vi "rszvl_core_global.vi"() -> ()   [LabVIEW 2014] (continued)
"Data Type"=4, "Access"=1, "Identifier"="RSZVL_ATTR_MARKER_SEARCH_PEAK", "Range Table"="", "Command"="CALC:MARK{Marker}:MAX", "Read Callback"="", "Write Callback"="", "Range Callback"="", "Check Callback"="", "Rngtable Callback"="", "Coerce Callback"="", "User Callback"="", "Supported Models"="", "Instrument Options"="", "Repeated Capabilities"="", "Restricted Repeated Capabilities"="", "Help"="This attribute positions the marker to the current maximum value of the corresponding trace. The corresponding marker is activated first or switched to the marker mode.\nNote: If no maximum value is found on the trace (level spacing to adjacent values < peak excursion), an execution error (error eode: -200) is produced.\n\nAvailable Repeated Capabilities:\nMarker: M1,M2,M3,M4\r\n\nRemote-control command(s):\nCALCulate<1|2>:MARKer<1 to 4>:MAXimum[:PEAK]", "Flags"={"OPC Wait"=FALSE, "Dont check status"=FALSE, "*WAI"=FALSE}, "Check Status Callback"=""}, {"Level"=3, "Descriptive Name"="Marker Search Peak Next Maximum", "Class Only"=FALSE, "Data Type"=4, "Access"=1, "Identifier"="RSZVL_ATTR_MARKER_SEARCH_PEAK_NEXT", "Range Table"="", "Command"="CALC:MARK{Marker}:MAX:NEXT", "Read Callback"="", "Write Callback"="", "Range Callback"="", "Check Callback"="", "Rngtable Callback"="", "Coerce Callback"="", "User Callback"="", "Supported Models"="", "Instrument Options"="", "Repeated Capabilities"="", "Restricted Repeated Capabilities"="", "Help"="This attribute positions the marker to the next smaller maximum value of the corresponding trace.\n\nNote: If no next smaller maximum value is found on the trace (level spacing to adjacent values < peak excursion), an execution error (error code: -200) is produced.\n\nAvailable Repeated Capabilities:\nMarker: M1,M2,M3,M4\r\n\nRemote-control command(s):\nCALCulate<1|2>:MARKer<1 to 4>:MAXimum:NEXT", "Flags"={"OPC Wait"=FALSE, "Dont check status"=FALSE, "*WAI"=FALSE}, "Check Status Callback"=""}, {"Level"=3, "Descriptive Name"="Marker Search Peak Right Maximum", "Class Only"=FALSE, "Data Type"=4, "Access"=1, "Identifier"="RSZVL_ATTR_MARKER_SEARCH_PEAK_RIGHT", "Range Table"="", "Command"="CALC:MARK{Marker}:MAX:RIGH", "Read Callback"="", "Write Callback"="", "Range Callback"="", "Check Callback"="", "Rngtable Callback"="", "Coerce Callback"="", "User Callback"="", "Supported Models"="", "Instrument Options"="", "Repeated Capabilities"="", "Restricted Repeated Capabilities"="", "Help"="This attribute positions the marker to the next smaller maximum value to the right of the current value (i.e. in ascending X values) on the corresponding trace.\n\nNote: If no next smaller maximum value is found on the trace (level spacing to adjacent values < peak excursion), an execution error (error code: -200) is produced.\n\nAvailable Repeated Capabilities:\nMarker: M1,M2,M3,M4\r\n\nRemote-control command(s):\nCALCulate<1|2>:MARKer<1 to 4>:MAXimum:RIGHt", "Flags"={"OPC Wait"=FALSE, "Dont check status"=FALSE, "*WAI"=FALSE}, "Check Status Callback"=""}, {"Level"=3, "Descriptive Name"="Marker Search Peak Left Maximum", "Class Only"=FALSE, "Data Type"=4, "Access"=1, "Identifier"="RSZVL_ATTR_MARKER_SEARCH_PEAK_LEFT", "Range Table"="", "Command"="CALC:MARK{Marker}:MAX:LEFT", "Read Callback"="", "Write Callback"="", "Range Callback"="", "Check Callback"="", "Rngtable Callback"="", "Coerce Callback"="", "User Callback"="", "Supported Models"="", "Instrument Options"="", "Repeated Capabilities"="", "Restricted Repeated Capabilities"="", "Help"="This attribute positions the marker to the next smaller maximum value to the left of the current value (i.e. in descending X values) on the trace.\n\nNote: If no next smaller maximum value is found on the trace (level spacing to adjacent values < peak excursion), an execution error (error code: -200) is produced.\n\nAvailable Repeated Capabilities:\nMarker: M1,M2,M3,M4\r\n\nRemote-control command(s):\nCALCulate<1|2>:MARKer<1 to 4>:MAXimum:LEFT", "Flags"={"OPC Wait"=FALSE, "Dont check status"=FALSE, "*WAI"=FALSE}, "Check Status Callback"=""}, {"Level"=3, "Descriptive Name"="Marker Search Peak Minimum", "Class Only"=FALSE, "Data Type"=4, "Access"=1, "Identifier"="RSZVL_ATTR_MARKER_SEARCH_MIN", "Range Table"="", "Command"="CALC:MARK{Marker}:MIN", "Read Callback"="", "Write Callback"="", "Range Callback"="", "Check Callback"="", "Rngtable Callback"="", "Coerce Callback"="", "User Callback"="", "Supported Models"="", "Instrument Options"="", "Repeated Capabilities"="", "Restricted Repeated Capabilities"="", "Help"="This attribute positions the marker to the current minimum value of the corresponding trace. The corresponding marker is activated first or switched to marker mode, if necessary.\n\nNote: If no minimum value is found on the trace (level spacing to adjacent values < peak excursion), an execution error (error code: -200) is produced.\n\nAvailable Repeated Capabilities:\nMarker: M1,M2,M3,M4\r\n\nRemote-control command(s):\nCALCulate<1|2>:MARKer<1 to 4>:MINimum[:PEAK]", "Flags"={"OPC Wait"=FALSE, "Dont check status"=FALSE, "*WAI"=FALSE}, "Check Status Callback"=""}, {"Level"=3, "Descriptive Name"="Marker Search Next Minimum", "Class Only"=FALSE, "Data Type"=4, "Access"=1, "Identifier"="RSZVL_ATTR_MARKER_SEARCH_MIN_NEXT", "Range Table"="", "Command"="CALC:MARK{Marker}:MIN:NEXT", "Read Callback"="", "Write Callback"="", "Range Callback"="", "Check Callback"="", "Rngtable Callback"="", "Coerce Callback"="", "User Callback"="", "Supported Models"="", "Instrument Options"="", "Repeated Capabilities"="", "Restricted Repeated Capabilities"="", "Help"="This attribute positions the marker to the next higher minimum value of the corresponding trace.\n\nNote: If no next higher minimum value is found on the trace (level spacing to adjacent values < peak excursion), an execution error (error code: -200) is produced.\n\nAvailable Repeated Capabilities:\nMarker: M1,M2,M3,M4\r\n\nRemote-control command(s):\nCALCulate<1|2>:MARKer<1 to 4>:MINimum:NEXT", "Flags"={"OPC Wait"=FALSE, "Dont check status"=FALSE, "*WAI"=FALSE}, "Check Status Callback"=""}, {"Level"=3, "Descriptive Name"="Marker Search Peak Maximum Auto", "Class Only"=FALSE, "Data Type"=3, "Access"=2, "Identifier"="RSZVL_ATTR_MARKER_SEARCH_PEAK_AUTO", "Range Table"="", "Command"="CALC:MARK:MAX:AUTO", "Read Callback"="", "Write Callback"="", "Range Callback"="", "Check Callback"="", "Rngtable Callback"="", "Coerce Callback"="", "User Callback"="", "Supported Models"="", "Instrument Options"="", "Repeated Capabilities"="", "Restricted Repeated Capabilities"="", "Help"="This attribute switches an automatic maximum peak search for marker 1 at the end of each particular sweep on and off. The actual marker search limit settings (LEFT LIMIT, RIGHT LIMIT, THRESHOLD, EXCLUDE LO) are taken into account.\n\nAvailable Repeated Capabilities:\nNone\n\nRemote-control command(s):\nCALCulate<1|2>:MARKer<1...4>:MAXimum:AUTO", "Flags"={"OPC Wait"=FALSE, "Dont check status"=FALSE, "*WAI"=FALSE}, "Check Status Callback"=""}, {"Level"=3, "Descriptive Name"="Marker Search Minimum Auto", "Class Only"=FALSE, "Data Type"=3, "Access"=2, "Identifier"="RSZVL_ATTR_MARKER_SEARCH_MIN_AUTO", "Range Table"="", "Command"="CALC:MARK:MIN:AUTO", "Read Callback"="", "Write Callback"="", "Range Callback"="", "Check Callback"="", "Rngtable Callback"="", "Coerce Callback"="", "User Callback"="", "Supported Models"="", "Instrument Options"="", "Repeated Capabilities"="", "Restricted Repeated Capabilities"="", "Help"="This attribute switches an automatic minimum peak search for marker 1 at the end of each particular sweep on and off. The actual marker search limit settings (LEFT LIMIT, RIGHT LIMIT, THRESHOLD, EXCLUDE LO) are taken into account.\n\nAvailable Repeated Capabilities:\nNone\n\nRemote-control command(s):\nCALCulate<1|2>:MARKer<1...4>:MINimum:AUTO", "Flags"={"OPC Wait"=FALSE, "Dont check status"=FALSE, "*WAI"=FALSE}, "Check Status Callback"=""}, {"Level"=2, "Descriptive Name"="Marker Search Configuration", "Class Only"=TRUE, "Data Type"=0, "Access"=0, "Identifier"="", "Range Table"="", "Command"="", "Read Callback"="", "Write Callback"="", "Range Callback"="", "Check Callback"="", "Rngtable Callback"="", "Coerce Callback"="", "User Callback"="", "Supported Models"="", "Instrument Options"="", "Repeated Capabilities"="", "Restricted Repeated Capabilities"="", "Help"="Configures marker search parameters.\n\n(1) Marker Threshold State:\nThis attribute switches on or off the threshold line. The unit depends on the setting performed with CALC:UNIT.\n\n(2) Marker Threshold:\nThis attribute defines the threshold value for the maximum/minimum search of markers with marker search functions MAX PEAK, NEXT PEAK, etc. The associated display line is automatically switched on.\n\n(3) Marker Peak Excursion:\nThis attribute defines the peak excursion., i.e. the spacing below a trace maximum which must be attained before a new maximum is recognized, or the spacing above a trace minimum which must be attained before a new minimum is recognized. The set value is valid for all markers and delta markers. The unit depends on the selected operating mode.\n\n(4) Marker Search Limits State:\nThis attribute switches between a limited (ON) and unlimited (OFF) search range. The function is independent of the selection of a marker.\n\n(5) Marker Search Limits Left:\nThis attribute sets the left limit of the search range for markers and delta markers. Depending on the x axis domain the indicated value defines a frequency (span > 0) or time (span = 0). The function is independent of the selection of a marker.\n\n(6) Marker Search Limits Right:\nThis attribute sets the right limit of the search range for markers and delta markers. Depending on the x axis domain the indicated value defines a frequency (span > 0) or time (span = 0). The function is independent of the selection of a marker.", "Flags"={"OPC Wait"=FALSE, "Dont check status"=FALSE, "*WAI"=FALSE}, "Check Status Callback"=""}, {"Level"=3, "Descriptive Name"="Marker Threshold State", "Class Only"=FALSE, "Data Type"=3, "Access"=2, "Identifier"="RSZVL_ATTR_MARKER_THRESHOLD_STATE", "Range Table"="", "Command"="CALC:THR:STAT", "Read Callback"="", "Write Callback"="", "Range Callback"="", "Check Callback"="", "Rngtable Callback"="", "Coerce Callback"="", "User Callback"="", "Supported Models"="", "Instrument Options"="", "Repeated Capabilities"="", "Restricted Repeated Capabilities"="", "Help"="This attribute switches on or off the threshold line. The unit depends on the setting performed with CALC:UNIT.\n\nAvailable Repeated Capabilities:\nNone\n\nRemote-control command(s):\nCALCulate<1|2>:THReshold:STATe ON | OFF", "Flags"={"OPC Wait"=FALSE, "Dont check status"=FALSE, "*WAI"=FALSE}, "Check Status Callback"=""}, {"Level"=3, "Descriptive Name"="Marker Threshold", "Class Only"=FALSE, "Data Type"=1, "Access"=2, "Identifier"="RSZVL_ATTR_MARKER_THRESHOLD", "Range Table"="", "Command"="CALC:THR", "Read Callback"="", "Write Callback"="", "Range Callback"="", "Check Callback"="", "Rngtable Callback"="", "Coerce Callback"="", "User Callback"="", "Supported Models"="", "Instrument Options"="", "Repeated Capabilities"="", "Restricted Repeated Capabilities"="", "Help"="This attribute defines the threshold value for the maximum/minimum search of markers with marker search functions MAX PEAK, NEXT PEAK, etc. The associated display line is automatically switched on.\n\nAvailable Repeated Capabilities:\nNone\n\nRemote-control command(s):\nCALCulate<1|2>:THReshold", "Flags"={"OPC Wait"=FALSE, "Dont check status"=FALSE, "*WAI"=FALSE}, "Check Status Callback"=""}, {"Level"=3, "Descriptive Name"="Marker Peak Excursion", "Class Only"=FALSE, "Data Type"=1, "Access"=2, "Identifier"="RSZVL_ATTR_PEAK_EXCURSION", "Range Table"="", "Command"="CALC:MARK:PEXC", "Read Callback"="", "Write Callback"="", "Range Callback"="", "Check Callback"="", "Rngtable Callback"="", "Coerce Callback"="", "User Callback"="", "Supported Models"="", "Instrument Options"="", "Repeated Capabilities"="", "Restricted Repeated Capabilities"="", "Help"="This attribute defines the peak excursion., i.e. the spacing below a trace maximum which must be attained before a new maximum is recognized, or the spacing above a trace minimum which must be attained before a new minimum is recognized. The set value is valid for all markers and delta markers. The unit depends on the selected operating mode.\n\nAvailable Repeated Capabilities:\nNone\n\nRemote-control command(s):\nCALCulate<1|2>:MARKer<1 to 4>:PEXCursion", "Flags"={"OPC Wait"=FALSE, "Dont check status"=FALSE, "*WAI"=FALSE}, "Check Status Callback"=""}, {"Level"=3, "Descriptive Name"="Marker Search Limits State", "Class Only"=FALSE, "Data Type"=3, "Access"=2, "Identifier"="RSZVL_ATTR_MARKER_SEARCH_LIMITS_STATE", "Range Table"="", "Command"="CALC:MARK:X:SLIM", "Read Callback"="", "Write Callback"="", "Range Callback"="", "Check Callback"="", "Rngtable Callback"="", "Coerce Callback"="", "User Callback"="", "Supported Models"="", "Instrument Options"="", "Repeated Capabilities"="", "Restricted Repeated Capabilities"="", "Help"="This attribute switches between a limited (ON) and unlimited (OFF) search range. The function is independent of the selection of a marker.\n\nAvailable Repeated Capabilities:\nNone\n\nRemote-control command(s):\nCALCulate<1|2>:MARKer<1 to 4>:X:SLIMits[:STATe] ON | OFF", "Flags"={"OPC Wait"=FALSE, "Dont check status"=FALSE, "*WAI"=FALSE}, "Check Status Callback"=""}, {"Level"=3, "Descriptive Name"="Marker Search Limits Left", "Class Only"=FALSE, "Data Type"=1, "Access"=2, "Identifier"="RSZVL_ATTR_MARKER_SEARCH_LIMITS_LEFT", "Range Table"="", "Command"="CALC:MARK:X:SLIM:LEFT", "Read Callback"="", "Write Callback"="", "Range Callback"="", "Check Callback"="", "Rngtable Callback"="", "Coerce Callback"="", "User Callback"="", "Supported Models"="", "Instrument Options"="", "Repeated Capabilities"="", "Restricted Repeated Capabilities"="", "Help"="This attribute sets the left limit of the search range for markers and delta markers. Depending on the x axis domain the indicated value defines a frequency (span > 0) or time (span = 0). The function is independent of the selection of a marker.\n\nAvailable Repeated Capabilities:\nNone\n\nRemote-control command(s):\nCALCulate<1|2>:MARKer<1 to 4>:X:SLIMits:LEFT", "Flags"={"OPC Wait"=FALSE, "Dont check status"=FALSE, "*WAI"=FALSE}, "Check Status Callback"=""}, {"Level"=3, "Descriptive Name"="Marker Search Limits Right", "Class Only"=FALSE, "Data Type"=1, "Access"=2, "Identifier"="RSZVL_ATTR_MARKER_SEARCH_LIMITS_RIGHT", "Range Table"="", "Command"="CALC:MARK:X:SLIM:RIGHT", "Read Callback"="", "Write Callback"="", "Range Callback"="", "Check Callback"="", "Rngtable Callback"="", "Coerce Callback"="", "User Callback"="", "Supported Models"="", "Instrument Options"="", "Repeated Capabilities"="", "Restricted Repeated Capabilities"="", "Help"="This attribute sets the right limit of the search range for markers and delta markers. Depending on the x axis domain the indicated value defines a frequency (span > 0) or time (span = 0). The function is independent of the selection of a marker.\n\nAvailable Repeated Capabilities:\nNone\n\nRemote-control command(s):\nCALCulate<1|2>:MARKer<1 to 4>:X:SLIMits:RIGHT", "Flags"={"OPC Wait"=FALSE, "Dont check status"=FALSE, "*WAI"=FALSE}, "Check Status Callback"=""}, {"Level"=2, "Descriptive Name"="Marker Functions", "Class Only"=TRUE, "Data Type"=0, "Access"=0, "Identifier"="", "Range Table"="", "Command"="", "Read Callback"="", "Write Callback"="", "Range Callback"="", "Check Callback"="", "Rngtable Callback"="", "Coerce Callback"="", "User Callback"="", "Supported Models"="", "Instrument Options"="", "Repeated Capabilities"="", "Restricted Repeated Capabilities"="", "Help"="Marker Functions.\n\n(1) Marker Peak List Count:\nThis attribute searches the selected trace for the indicated number of maxima. The number of maxima found depends on the waveform and value set for the Peak Excursion parameter, however, a maximum number of 50 maxima are determined. Only the signals which exceed their surrounding values at least by the value indicated by the peak excursion parameter will be recognized as maxima. Therefore, the number of maxima found is not automatically the same as the number of maxima desired.\n\n(2) Marker Peak List Found:\nThis attribute reads out the number of maxima found during the search. If no search for maxima has been performed, 0 is returned.\n\n(3) Marker Peak List Sort:\nThis attribute sets the sort mode for the search for maxima.\n\n(4) Marker Zoom:\nThis attribute defines the range to be zoomed around marker 1. Marker 1 is activated first, if necessary.\nThe subsequent frequency sweep is stopped at the marker position and the frequency of the signal is counted. This frequency becomes the new center frequency, and the zoomed span is set. In order to recognize the end of the operation the synchronization to the sweep end should be activated. This is only possible in single sweep mode.\n\n(5) Marker Demodulation State:\nThis attribute switches on or off the audio demodulator when the indicated marker is reached. In the frequency domain (span > 0) the hold time can be defined at the corresponding marker position with RSZVL_ATTR_MARKER_DEMOD_HOLDOFF.\nIn the time domain (span = 0) the demodulation is permanently active.\n\n(6) Marker Demodulation Type:\nThis attribute selects the demodulation type for the audio demodulator.\n\n(7) Marker Demodulation Holdoff:\nThis attribute defines the hold time at the marker position for the demodulation in the frequency domain (span > 0).\n\n(8) Marker Demodulation Continuous:\nThis attribute switches on or off the continuous demodulation in the frequency domain (span >0). Thus acoustic monitoring of the signals can be performed in the frequency domain. The function does not depend on the selected marker.\n\n(9) Marker To Center:\nThis attribute sets the center frequency equal to the frequency of the indicated marker.\nIf marker 2, 3 or 4 is selected and used as delta marker, it is switched to the marker mode.\n\n(10) Marker To Step Width:\nThis attribute sets the step width of the center frequency to the X value of the current marker. If marker 2, 3 or 4 is selected and used as delta marker, it is switched to the marker mode.\n\n(11) Marker To Reference:\nThis attribute sets the reference level to the power measured by the indicated marker. If marker 2, 3 or 4 is selected and used as delta marker, it is switched to marker mode.\n\n(12) Marker Fixed Reference State:\nThis attribute switches the relative measurement to a fixed reference value on or off. Marker 1 will be activated previously and a peak search will be performed, if necessary. If marker 1 is activated, its position becomes the reference point for the measurement. The reference point can then be modified with commands CALCulate:DELTamarker:FUNCtion:FIXed:RPOint:X and to :RPOint:Y independently of the position of marker 1 and of a trace. It is valid for all delta markers as long as the function is active.\n\n(13) Marker Fixed Ref Point Level:\nThis attribute defines a new reference point level for all delta markers for a measurement with fixed reference point.\n(CALCulate:DELTamarker:FUNCtion:FIXed:STATe ON).\nFor phase-noise measurements (CALCulate:DELTamarker:FUNCtion:PNOise:STATe ON), the command defines a new reference point level for delta marker 2.\n\n(14) Marker Fixed Ref Point Level Offset:\nThis attribute defines an additional level offset for the measurement with fixed reference value (CALCulate:DELTamarker:FUNCtion:FIXed:STATe ON). For this measurement, the offset is included in the display of all delta markers.\nFor phase-noise measurements (CALCulate:DELTamarker:FUNCtion:PNOise:STATe ON), the command defines an additional level offset which is included in the display of delta marker 2.\n\n(15) Marker Fixed Ref Point Frequency:\nThis attribute defines a new reference frequency (span > 0) or time (span = 0) for all delta markers for a measurement with fixed reference value (CALCulate:DELTamarker:FUNCtion:FIXed:STATe ON).\nFor phase-noise measurements (CALCulate:DELTamarker:FUNCtion:PNOise:STATe ON), the command defines a new reference frequency or time for delta marker 2.\n\n(16) Marker Fixed Ref Point Peak Search:\nThis attribute sets the reference point level for all delta markers for a measurement with fixed reference point (CALC:DELT:FUNC:FIX:STAT ON) to the peak of the selected trace.", "Flags"={"OPC Wait"=FALSE, "Dont check status"=FALSE, "*WAI"=FALSE}, "Check Status Callback"=""}, {"Level"=3, "Descriptive Name"="Marker Peak List Count", "Class Only"=FALSE, "Data Type"=0, "Access"=2, "Identifier"="RSZVL_ATTR_MARKER_PEAK_LIST_COUNT", "Range Table"="rszvl_rngMarkerPeakListCount", "Command"="CALC:MARK{Marker}:FUNC:FPE", "Read Callback"="", "Write Callback"="", "Range Callback"="", "Check Callback"="", "Rngtable Callback"="", "Coerce Callback"="", "User Callback"="", "Supported Models"="", "Instrument Options"="", "Repeated Capabilities"="", "Restricted Repeated Capabilities"="", "Help"="This attribute searches the selected trace for the indicated number of maxima. The number of maxima found depends on the waveform and value set for the Peak Excursion parameter, however, a maximum number of 50 maxima are determined. Only the signals which exceed their surrounding values at least by the value indicated by the peak excursion parameter will be recognized as maxima. Therefore, the number of maxima found is not automatically the same as the number of maxima desired.\n\nAvailable Repeated Capabilities:\nMarker: M1,M2,M3,M4\r\n\nRemote-control command(s):\nCALCulate<1|2>:MARKer<1 to 4>:FUNCtion:FPEaks[:IMMediate]", "Flags"={"OPC Wait"=FALSE, "Dont check status"=FALSE, "*WAI"=FALSE}, "Check Status Callback"=""}, {"Level"=3, "Descriptive Name"="Marker Peak List Found", "Class Only"=FALSE, "Data Type"=0, "Access"=0, "Identifier"="RSZVL_ATTR_MARKER_PEAK_LIST_FOUND", "Range Table"="", "Command"="CALC:MARK{Marker}:FUNC:FPE:COUN?", "Read Callback"="", "Write Callback"="", "Range Callback"="", "Check Callback"="", "Rngtable Callback"="", "Coerce Callback"="", "User Callback"="", "Supported Models"="", "Instrument Options"="", "Repeated Capabilities"="", "Restricted Repeated Capabilities"="", "Help"="This attribute reads out the number of maxima found during the search. If no search for maxima has been performed, 0 is returned.\n\nAvailable Repeated Capabilities:\nMarker: M1,M2,M3,M4\r\n\nRemote-control command(s):\nCALCulate<1|2>:MARKer<1 to 4>:FUNCtion:FPEaks:COUNt?", "Flags"={"OPC Wait"=FALSE, "Dont check status"=FALSE, "*WAI"=FALSE}, "Check Status Callback"=""}, {"Level"=3, "Descriptive Name"="Marker Peak List Sort", "Class Only"=FALSE, "Data Type"=0, "Access"=2, "Identifier"="RSZVL_ATTR_MARKER_PEAK_LIST_SORT", "Range Table"="rszvl_rngMarkerPeakListSort", "Command"="CALC:MARK{Marker}:FUNC:FPE:SORT", "Read Callback"="", "Write Callback"="", "Range Callback"="", "Check Callback"="", "Rngtable Callback"="", "Coerce Callback"="", "User Callback"="", "Supported Models"="", "Instrument Options"="", "Repeated Capabilities"="", "Restricted Repeated Capabilities"="", "Help"="This attribute sets the sort mode for the search for maxima.\n\nAvailable Repeated Capabilities:\nMarker: M1,M2,M3,M4\r\n\nRemote-control command(s):\nCALCulate<1|2>:MARKer<1 to 4>:FUNCtion:FPEaks:SORT X | Y", "Flags"={"OPC Wait"=FALSE, "Dont check status"=FALSE, "*WAI"=FALSE}, "Check Status Callback"=""}, {"Level"=3, "Descriptive Name"="Marker Zoom", "Class Only"=FALSE, "Data Type"=1, "Access"=2, "Identifier"="RSZVL_ATTR_MARKER_ZOOM", "Range Table"="", "Command"="CALC:MARK:FUNC:ZOOM", "Read Callback"="", "Write Callback"="", "Range Callback"="", "Check Callback"="", "Rngtable Callback"="", "Coerce Callback"="", "User Callback"="", "Supported Models"="", "Instrument Options"="", "Repeated Capabilities"="", "Restricted Repeated Capabilities"="", "Help"="This attribute defines the range to be zoomed around marker 1. Marker 1 is activated first, if necessary.\nThe subsequent frequency sweep is stopped at the marker position and the frequency of the signal is counted. This frequency becomes the new center frequency, and the zoomed span is set. In order to recognize the end of the operation the synchronization to the sweep end should be activated. This is only possible in single sweep mode.\n\nAvailable Repeated Capabilities:\nNone\n\nRemote-control command(s):\nCALCulate<1|2>:MARKer<1 to 4>:FUNCtion:ZOOM", "Flags"={"OPC Wait"=TRUE, "Dont check status"=FALSE, "*WAI"=FALSE}, "Check Status Callback"=""}, {"Level"=3, "Descriptive Name"="Marker Demodulation State", "Class Only"=FALSE, "Data Type"=3, "Access"=2, "Identifier"="RSZVL_ATTR_MARKER_DEMOD_STATE", "Range Table"="", "Command"="CALC:MARK{Marker}:FUNC:DEM", "Read Callback"="", "Write Callback"="", "Range Callback"="", "Check Callback"="", "Rngtable Callback"="", "Coerce Callback"="", "User Callback"="", "Supported Models"="", "Instrument Options"="", "Repeated Capabilities"="", "Restricted Repeated Capabilities"="", "Help"="This attribute switches on or off the audio demodulator when the indicated marker is reached. In the frequency domain (span > 0) the hold time can be defined at the corresponding marker position with RSZVL_ATTR_MARKER_DEMOD_HOLDOFF.\nIn the time domain (span = 0) the demodulation is permanently active.\n\nAvailable Repeated Capabilities:\nMarker: M1,M2,M3,M4\r\n\nRemote-control command(s):\nCALCulate<1|2>:MARKer<1 to 4>:FUNCtion:DEModulation[:STATe] ON | OFF", "Flags"={"OPC Wait"=FALSE, "Dont check status"=FALSE, "*WAI"=FALSE}, "Check Status Callback"=""}, {"Level"=3, "Descriptive Name"="Marker Demodulation Type", "Class Only"=FALSE, "Data Type"=0, "Access"=2, "Identifier"="RSZVL_ATTR_MARKER_DEMOD_TYPE", "Range Table"="rszvl_rngMarkerDemodType", "Command"="CALC:MARK:FUNC:DEM:SEL", "Read Callback"="", "Write Callback"="", "Range Callback"="", "Check Callback"="", "Rngtable Callback"="", "Coerce Callback"="", "User Callback"="", "Supported Models"="", "Instrument Options"="", "Repeated Capabilities"="", "Restricted Repeated Capabilities"="", "Help"="This attribute selects the demodulation type for the audio demodulator.\n\nAvailable Repeated Capabilities:\nNone\n\nRemote-control command(s):\nCALCulate<1|2>:MARKer<1 to 4>:FUNCtion:DEModulation:SELect AM | FM", "Flags"={"OPC Wait"=FALSE, "Dont check status"=FALSE, "*WAI"=FALSE}, "Check Status Callback"=""}, {"Level"=3, "Descriptive Name"="Marker Demodulation Holdoff", "Class Only"=FALSE, "Data Type"=1, "Access"=2, "Identifier"="RSZVL_ATTR_MARKER_DEMOD_HOLDOFF", "Range Table"="rszvl_rngMarkerDemodHoldoff", "Command"="CALC:MARK:FUNC:DEM:HOLD", "Read Callback"="", "Write Callback"="", "Range Callback"="", "Check Callback"="", "Rngtable Callback"="", "Coerce Callback"="", "User Callback"="", "Supported Models"="", "Instrument Options"="", "Repeated Capabilities"="", "Restricted Repeated Capabilities"="", "Help"="This attribute defines the hold time at the marker position for the demodulation in the frequency domain (span > 0).\n\nAvailable Repeated Capabilities:\nNone\n\nRemote-control command(s):\nCALCulate<1|2>:MARKer<1 to 4>:FUNCtion:DEModulation:HOLDoff", "Flags"={"OPC Wait"=FALSE, "Dont check status"=FALSE, "*WAI"=FALSE}, "Check Status Callback"=""}, {"Level"=3, "Descriptive Name"="Marker Demodulation Continuous", "Class Only"=FALSE, "Data Type"=3, "Access"=2, "Identifier"="RSZVL_ATTR_MARKER_DEMOD_CONT", "Range Table"="", "Command"="CALC:MARK:FUNC:DEM:CONT", "Read Callback"="", "Write Callback"="", "Range Callback"="", "Check Callback"="", "Rngtable Callback"="", "Coerce Callback"="", "User Callback"="", "Supported Models"="", "Instrument Options"="", "Repeated Capabilities"="", "Restricted Repeated Capabilities"="", "Help"="This attribute switches on or off the continuous demodulation in the frequency domain (span >0). Thus acoustic monitoring of the signals can be performed in the frequency domain. The function does not depend on the selected marker.\n\nAvailable Repeated Capabilities:\nNone\n\nRemote-control command(s):\nCALCulate<1|2>:MARKer<1 to 4>:FUNCtion:DEModulation:CONTinuous ON | OFF", "Flags"={"OPC Wait"=FALSE, "Dont check status"=FALSE, "*WAI"=FALSE}, "Check Status Callback"=""}, {"Level"=3, "Descriptive Name"="Marker To Center", "Class Only"=FALSE, "Data Type"=4, "Access"=1, "Identifier"="RSZVL_ATTR_MARKER_TO_CENTER", "Range Table"="", "Command"="CALC:MARK{Marker}:FUNC:CENT", "Read Callback"="", "Write Callback"="", "Range Callback"="", "Check Callback"="", "Rngtable Callback"="", "Coerce Callback"="", "User Callback"="", "Supported Models"="", "Instrument Options"="", "Repeated Capabilities"="", "Restricted Repeated Capabilities"="", "Help"="This attribute sets the center frequency equal to the frequency of the indicated marker.\nIf marker 2, 3 or 4 is selected and used as delta marker, it is switched to the marker mode.\n\nAvailable Repeated Capabilities:\nMarker: M1,M2,M3,M4\r\n\nRemote-control command(s):\nCALCulate<1|2>:MARKer<1 to 4>:FUNCtion:CENTer", "Flags"={"OPC Wait"=FALSE, "Dont check status"=FALSE, "*WAI"=FALSE}, "Check Status Callback"=""}, {"Level"=3, "Descriptive Name"="Marker To Step Width", "Class Only"=FALSE, "Data Type"=4, "Access"=1, "Identifier"="RSZVL_ATTR_MARKER_TO_STEP", "Range Table"="", "Command"="CALC:MARK{Marker}:FUNC:CST", "Read Callback"="", "Write Callback"="", "Range Callback"="", "Check Callback"="", "Rngtable Callback"="", "Coerce Callback"="", "User Callback"="", "Supported Models"="", "Instrument Options"="", "Repeated Capabilities"="", "Restricted Repeated Capabilities"="", "Help"="This attribute sets the step width of the center frequency to the X value of the current marker. If marker 2, 3 or 4 is selected and used as delta marker, it is switched to the marker mode.\n\nAvailable Repeated Capabilities:\nMarker: M1,M2,M3,M4\r\n\nRemote-control command(s):\nCALCulate<1|2>:MARKer<1 to 4>:FUNCtion:CSTep", "Flags"={"OPC Wait"=FALSE, "Dont check status"=FALSE, "*WAI"=FALSE}, "Check Status Callback"=""}, {"Level"=3, "Descriptive Name"="Marker To Reference", "Class Only"=FALSE, "Data Type"=4, "Access"=1, "Identifier"="RSZVL_ATTR_MARKER_TO_REFERENCE", "Range Table"="", "Command"="CALC:MARK{Marker}:FUNC:REF", "Read Callback"="", "Write Callback"="", "Range Callback"="", "Check Callback"="", "Rngtable Callback"="", "Coerce Callback"="", "User Callback"="", "Supported Models"="", "Instrument Options"="", "Repeated Capabilities"="", "Restricted Repeated Capabilities"="", "Help"="This attribute sets the reference level to the power measured by the indicated marker. If marker 2, 3 or 4 is selected and used as delta marker, it is switched to marker mode.\n\nAvailable Repeated Capabilities:\nMarker: M1,M2,M3,M4\r\n\nRemote-control command(s):\nCALCulate<1|2>:MARKer<1 to 4>:FUNCtion:REFerence", "Flags"={"OPC Wait"=FALSE, "Dont check status"=FALSE, "*WAI"=FALSE}, "Check Status Callback"=""}, {"Level"=3, "Descriptive Name"="Marker Fixed Reference State", "Class Only"=FALSE, "Data Type"=3, "Access"=2, "Identifier"="RSZVL_ATTR_MARKER_REF_STATE", "Range Table"="", "Command"="CALC:DELT:FUNC:FIX", "Read Callback"="", "Write Callback"="", "Range Callback"="", "Check Callback"="", "Rngtable Callback"="", "Coerce Callback"="", "User Callback"="", "Supported Models"="", "Instrument Options"="", "Repeated Capabilities"="", "Restricted Repeated Capabilities"="", "Help"="This attribute switches the relative measurement to a fixed reference value on or off. Marker 1 will be activated previously and a peak search will be performed, if necessary. If marker 1 is activated, its position becomes the reference point for the measurement. The reference point can then be modified with commands CALCulate:DELTamarker:FUNCtion:FIXed:RPOint:X and to :RPOint:Y independently of the position of marker 1 and of a trace. It is valid for all delta markers as long as the function is active.\n\nAvailable Repeated Capabilities:\nNone\n\nRemote-control command(s):\nCALCulate<1|2>:DELTamarker<1 to 4>:FUNCtion:FIXed[:STATe] ON | OFF", "Flags"={"OPC Wait"=FALSE, "Dont check status"=FALSE, "*WAI"=FALSE}, "Check Status Callback"=""}, {"Level"=3, "Descriptive Name"="Marker Fixed Ref Point Level", "Class Only"=FALSE, "Data Type"=1, "Access"=2, "Identifier"="RSZVL_ATTR_MARKER_REF_LEVEL", "Range Table"="rszvl_rngRefLevel", "Command"="CALC:DELT:FUNC:FIX:RPO:Y", "Read Callback"="", "Write Callback"="", "Range Callback"="", "Check Callback"="", "Rngtable Callback"="", "Coerce Callback"="", "User Callback"="", "Supported Models"="", "Instrument Options"="", "Repeated Capabilities"="", "Restricted Repeated Capabilities"="", "Help"="This attribute defines a new reference point level for all delta markers for a measurement with fixed reference point.\n(CALCulate:DELTamarker:FUNCtion:FIXed:STATe ON).\nFor phase-noise measurements (CALCulate:DELTamarker:FUNCtion:PNOise:STATe ON), the command defines a new reference point level for delta marker 2.\n\nAvailable Repeated Capabilities:\nNone\n\nRemote-control command(s):\nCALCulate<1|2>:DELTamarker<1 to 4>:FUNCtion:FIXed:RPOint:Y", "Flags"={"OPC Wait"=FALSE, "Dont check status"=FALSE, "*WAI"=FALSE}, "Check Status Callback"=""}, {"Level"=3, "Descriptive Name"="Marker Fixed Ref Point Level Offset", "Class Only"=FALSE, "Data Type"=1, "Access"=2, "Identifier"="RSZVL_ATTR_MARKER_REF_LEVEL_OFFSET", "Range Table"="rszvl_rngRefLevelOffset", "Command"="CALC:DELT:FUNC:FIX:RPO:Y:OFFS", "Read Callback"="", "Write Callback"="", "Range Callback"="", "Check Callback"="", "Rngtable Callback"="", "Coerce Callback"="", "User Callback"="", "Supported Models"="", "Instrument Options"="", "Repeated Capabilities"="", "Restricted Repeated Capabilities"="", "Help"="This attribute defines an additional level offset for the measurement with fixed reference value (CALCulate:DELTamarker:FUNCtion:FIXed:STATe ON). For this measurement, the offset is included in the display of all delta markers.\nFor phase-noise measurements (CALCulate:DELTamarker:FUNCtion:PNOise:STATe ON), the command defines an additional level offset which is included in the display of delta marker 2.\n\nAvailable Repeated Capabilities:\nNone\n\nRemote-control command(s):\nCALCulate<1|2>:DELTamarker<1 to 4>:FUNCtion:FIXed:RPOint:Y:OFFSet", "Flags"={"OPC Wait"=FALSE, "Dont check status"=FALSE, "*WAI"=FALSE}, "Check Status Callback"=""}, {"Level"=3, "Descriptive Name"="Marker Fixed Ref Point Frequency", "Class Only"=FALSE, "Data Type"=1, "Access"=2, "Identifier"="RSZVL_ATTR_MARKER_REF_FREQ", "Range Table"="", "Command"="CALC:DELT:FUNC:FIX:RPO:X", "Read Callback"="", "Write Callback"="", "Range Callback"="", "Check Callback"="", "Rngtable Callback"="", "Coerce Callback"="", "User Callback"="", "Supported Models"="", "Instrument Options"="", "Repeated Capabilities"="", "Restricted Repeated Capabilities"="", "Help"="This attribute defines a new reference frequency (span > 0) or time (span = 0) for all delta markers for a measurement with fixed reference value (CALCulate:DELTamarker:FUNCtion:FIXed:STATe ON).\nFor phase-noise measurements (CALCulate:DELTamarker:FUNCtion:PNOise:STATe ON), the command defines a new reference frequency or time for delta marker 2.\n\nAvailable Repeated Capabilities:\nNone\n\nRemote-control command(s):\nCALCulate<1|2>:DELTamarker<1 to 4>:FUNCtion:FIXed:RPOint:X", "Flags"={"OPC Wait"=FALSE, "Dont check status"=FALSE, "*WAI"=FALSE}, "Check Status Callback"=""}, {"Level"=3, "Descriptive Name"="Marker Fixed Ref Point Peak Search", "Class Only"=FALSE, "Data Type"=4, "Access"=1, "Identifier"="RSZVL_ATTR_MARKER_REF_PEAK", "Range Table"="", "Command"="CALC:DELT:FUNC:FIX:RPO:MAX", "Read Callback"="", "Write Callback"="", "Range Callback"="", "Check Callback"="", "Rngtable Callback"="", "Coerce Callback"="", "User Callback"="", "Supported Models"="", "Instrument Options"="", "Repeated Capabilities"="", "Restricted Repeated Capabilities"="", "Help"="This attribute sets the reference point level for all delta markers for a measurement with fixed reference point (CALC:DELT:FUNC:FIX:STAT ON) to the peak of the selected trace.\n\nAvailable Repeated Capabilities:\nNone\n\nRemote-control command(s):\nCALCulate<1|2>:DELTamarker<1 to 4>:FUNCtion:FIXed:RPOint:MAXimum[:PEAK]", "Flags"={"OPC Wait"=FALSE, "Dont check status"=FALSE, "*WAI"=FALSE}, "Check Status Callback"=""}, {"Level"=2, "Descriptive Name"="Delta Marker", "Class Only"=TRUE, "Data Type"=0, "Access"=0, "Identifier"="", "Range Table"="", "Command"="", "Read Callback"="", "Write Callback"="", "Range Callback"="", "Check Callback"="", "Rngtable Callback"="", "Coerce Callback"="", "User Callback"="", "Supported Models"="", "Instrument Options"="", "Repeated Capabilities"="", "Restricted Repeated Capabilities"="", "Help"="Delta Marker attributes configuration.\n\n(1) Delta Marker State:\nThis attribute switches on and off the delta marker when delta marker 1 is selected. The corresponding marker becomes the delta marker when delta marker 2 to 4 is selected. If the corresponding marker is not activated, it will be activated and positioned on  the maximum of the measurement curve.\n\n(2) Delta Marker Mode:\nThis attribute switches between relative and absolute frequency input of the delta marker (or time with span = 0). It affects all delta markers.\nRepeated capabilitiy Delta Marker are used to prevent switching On Delta Marker 1, if the user uses Delta Marker 2.\n\n(3) Delta Marker Position:\nThis attribute positions the selected delta marker to the indicated frequency (span > 0), time (span = 0) or level (APD measurement = ON or CCDFmeasurement = ON). The input is in absolute values or relative to marker 1 depending on the attribute RSZVL_ATTR_REFERENCE_MARKER_MODE. If Reference Fixed measurement (CALCulate:DELTamarker:FUNCtion:FIXed:STATe ON) is active, relative values refer to the reference position are entered. The query always returns absolute values.\n\n(4) Delta Marker Relative Position:\nThis attribute queries the frequency (span > 0) or time (span = 0) of the selected delta marker relative to marker 1 or to the reference position ( for CALCulate:DELTamarker:FUNCtion:FIXed:STATe ON). The attribute activates the corresponding delta marker, if necessary.\n\n(5) Delta Marker Amplitude:\nThis attribute queries the measured value of the selected delta marker. The corresponding delta marker will be activated, if necessary. The output is always a relative value referred to marker 1 or to the reference position (reference fixed active).\n\n(6) Delta Marker Assign Trace:\nThis attribute assigns the selected delta marker to the indicated measurement curve. The selected measurement curve must be active, i.e. its state must be different from BLANK.\n\n(7) Delta Marker All Off:\nThis attribute switches off all active delta markers (screen A or screen B).", "Flags"={"OPC Wait"=FALSE, "Dont check status"=FALSE, "*WAI"=FALSE}, "Check Status Callback"=""}, {"Level"=3, "Descriptive Name"="Delta Marker State", "Class Only"=FALSE, "Data Type"=3, "Access"=2, "Identifier"="RSZVL_ATTR_REFERENCE_MARKER_STATE", "Range Table"="", "Command"="CALC:DELT{DeltaMarker}", "Read Callback"="", "Write Callback"="", "Range Callback"="", "Check Callback"="", "Rngtable Callback"="", "Coerce Callback"="", "User Callback"="", "Supported Models"="", "Instrument Options"="", "Repeated Capabilities"="", "Restricted Repeated Capabilities"="", "Help"="This attribute switches on and off the delta marker when delta marker 1 is selected. The corresponding marker becomes the delta marker when delta marker 2 to 4 is selected. If the corresponding marker is not activated, it will be activated and positioned on  the maximum of the measurement curve.\n\nAvailable Repeated Capabilities:\nDeltaMarker: DM1,DM2,DM3,DM4\r\n\nRemote-control command(s):\nCALCulate<1|2>:DELTamarker<1 to 4>[:STATe] ON | OFF"
